vi "sub_binary_pixel-sum.vi"(11 "image buff":T1) -> (2 "per":dbl, 3 "웨이브폼 차트":cluster{u64, u64}(graph))   [LabVIEW 2019]
uses:
  <vilib>/vision/Image Controls.llb/IMAQ Image.ctl
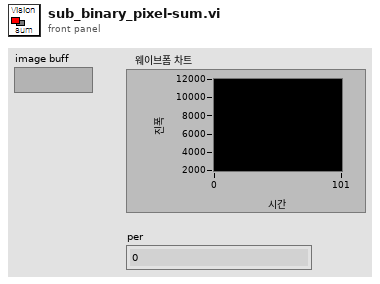
[diagram p1: front panel]
types:
  T1 = typedef "IMAQ Image.ctl" = refnum<image>
  T2 = cluster{"Global Rectangle":i32[], "Contours":cluster{"Contour Type":u32, "ROI Type":u32, "Points":i32[]}[]}
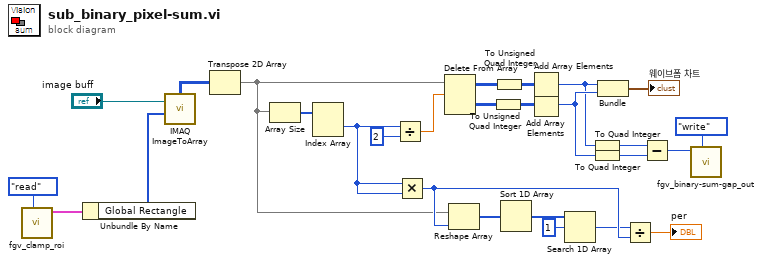
[diagram p0: block diagram]
diagram:
  n1 = call "fgv_clamp_roi.vi"("cmd"=enum16{"init", "read", "write"}."read") -> ("ROI-clamp out"=w3:T2)  [unwired: 10 in]
  n2 = Unbundle By Name(w3) -> ("Global Rectangle"=w4:i32[])
  n3 = call "IMAQ ImageToArray"("Optional Rectangle"=w4, "Image"="image buff") -> ("Image Pixels (U8)"=w12:u8[][])  [unwired: 2 in, 4 out]
  n4 = Transpose 2D Array(2D array=w12) -> (transposed array=w20:u8[][])
  n5 = Array Size(array=w20) -> (size(s)=w5:i32[])
  n6 = Index Array(array=w5) -> (element #1=w21:i32)  [unwired: 2 in, 1 out]
  n7 = Divide(x=w21, y=2) -> (x/y=w7:dbl)
  n8 = Multiply(x=w21, y=w21) -> (x*y=w26:i32)
  n9 = Delete From Array(array=w20, length=w7) -> (deleted portion=w9:u8[][], array with subset deleted=w8:u8[][])  [unwired: 2 in]
  n10 = Reshape Array(w20, w26) -> (w22:u8[])
  n11 = To Unsigned Quad Integer(1:w9) -> (0:w10:u64[][])
  n12 = To Unsigned Quad Integer(1:w8) -> (0:w11:u64[][])
  n13 = Sort 1D Array(array=w22) -> (sorted array=w23:u8[])
  n14 = Add Array Elements(numeric array=w11) -> (sum=w13:u64)
  n15 = Add Array Elements(numeric array=w10) -> (sum=w14:u64)
  n16 = Search 1D Array(1D array=w23, element=u8 1 ("원소")) -> (index of element=w25:i32)  [unwired: 1 in]
  n17 = To Quad Integer(1:w13) -> (0:w16:i64)
  n18 = To Quad Integer(1:w14) -> (0:w17:i64)
  n19 = Bundle(w13, w14) -> (→"웨이브폼 차트":cluster{u64, u64})  [unwired: 1 in]
  n20 = Divide(x=w25, y=w26) -> (x/y=→"per":dbl)
  n21 = Subtract(x=w16, y=w17) -> (x-y=w15:i64)
  n22 = call "fgv_binary-sum-gap_out.vi"("cmd"=enum16{"read", "write"}."write", "binary sum gap"=w15) -> ()  [unwired: 9 in, 1 out]
